vi "onHttpHead.vi"(6 "timeout":i32=10000, 8 "error in":errorcluster, 10 "url":string, 11 "http-method in":refnum<class "REST Client.lvclass">) -> (0 "error out":errorcluster, 2 "headers":string, 3 "http-method out":refnum<class "REST Client.lvclass">)   [LabVIEW 2020, in "REST Client.lvlib" / "REST Client.lvclass"]
uses:
  REST Client.lvclass
  REST Client.lvclass/REST Client.ctl
  http-client/http-client.lvclass
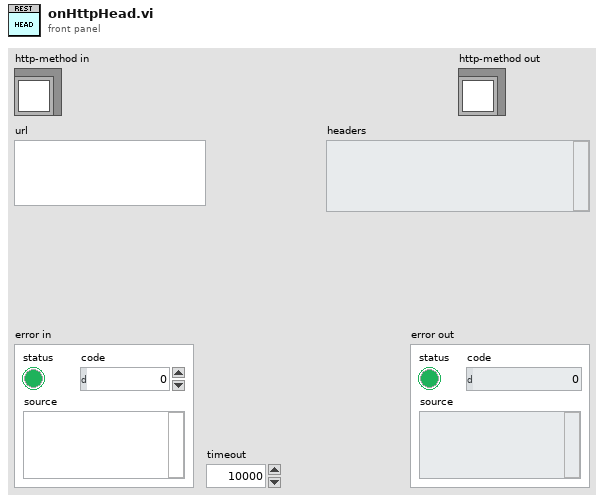
[diagram p1: front panel]
types:
  T1 = typedef "REST Client.lvlib/REST Client.lvclass/HTTP Header.ctl" = cluster{"header":T2, "value":string}
  T2 = typedef "lib_NI_Advanced HTTP Client.lvlib/Session.lvclass/Header--Combo Box.ctl" = string
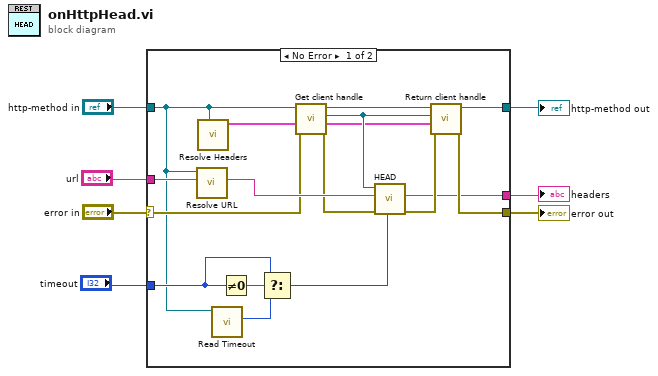
[diagram p0: block diagram]
diagram:
  n1 = case shown="No Error" "error in" {
    selector: "error in" -> [w13 w26]
    tunnel: [w9 w26] -> w1
    tunnel: [w10 w25] -> w2
    tunnel: "http-method in" -> [w12 w25]
    tunnel: "url" -> [w21 _]
    tunnel: "timeout" -> [w18 _]
    tunnel: [w8 _] -> w3
    frame No Error {
      n2 = call "Resolve URL.vi"("Path"=w21, "REST Client in"=w12) -> ("Resolved URL"=w20:string)  [unwired: 9 in]
      n3 = call "Resolve Headers.vi"("REST Client in"=w12) -> ("headers out"=w11:T1[])  [unwired: 10 in]
      n4 = call-dynamic "Read Timeout.vi"("REST Client in"=w12) -> ("Timeout"=w15:i32)  [unwired: 8 in, 2 out]
      n5 = Not Equal To 0?(x=w18) -> (x != 0?=w19:bool)
      n6 = Select(t=w18, s=w19, f=w15) -> (s? t:f=w17:i32)
      n7 = call "Get client handle.vi"("error in (no error)"=w13, "headers"=w11, "REST Client in"=w12) -> ("error out"=w16:errorcluster, "headers out"=w22:T1[], "http-client"=w23:refnum<class "http-client.lvclass">, "REST Client out"=w24:refnum<class "REST Client.lvclass">)  [unwired: 5 in]
      n8 = call "HEAD.vi"("timeout"=w17, "error in"=w16, "url"=w20, "http-client in"=w23) -> ("error out"=w14:errorcluster, "headers"=w8:string)  [unwired: 4 in, 2 out]
      n9 = call "Return client handle.vi"("error in (no error)"=w14, "headers"=w22, "http-client"=w23, "REST Client in"=w24) -> ("error out"=w9:errorcluster, "REST Client out"=w10:refnum<class "REST Client.lvclass">)  [unwired: 6 in]
    }
    frame Error {
    }
  }
  "error out" <- w1
  "http-method out" <- w2
  "headers" <- w3
